vi "fgv_calibrationPos_LBVals.vi"(7 "ACtions":enum16{"Initialise", "Get", "Set"}(ring), 8 "error in (no error)":errorcluster, 11 "Calibration Pos LBVals IN":string[][](array[string])) -> (0 "error out":errorcluster, 3 "Calibration Pos LBVals  OUT":string[][](array[string]))   [LabVIEW 2020]
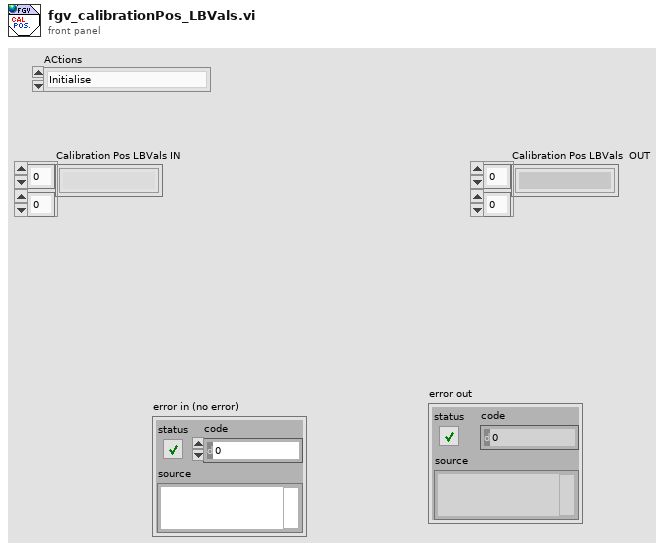
[diagram p1: front panel]
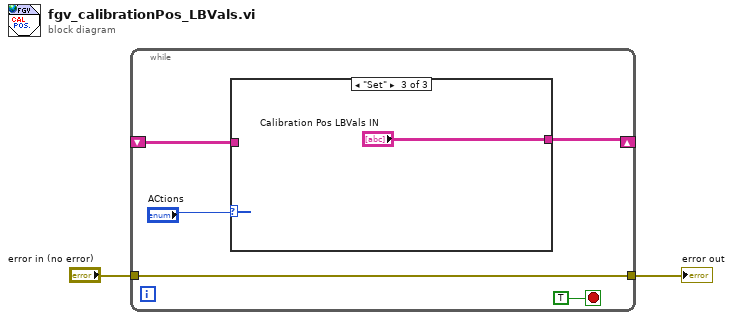
[diagram p0: block diagram]
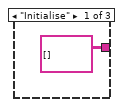
[diagram p2: hidden frame]
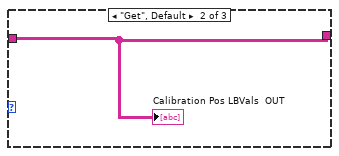
[diagram p3: hidden frame]
diagram:
  n1 = while {
    shift-right: [w6] -> _
    shift-left: _ -> [w5]
    tunnel: "error in (no error)" -> [w4]
    tunnel: [w4] -> w1
    stop <- TRUE stop-if-true
    n2 = case shown="\"Set\"" "ACtions" {
      tunnel: [string[][] [] ("Calibration Pos LBVals IN") w9 "Calibration Pos LBVals IN"] -> w6
      tunnel: w5 -> [_ w9 _]
      frame "Initialise" {
      }
      frame "Get", Default {
        "Calibration Pos LBVals  OUT" <- w9
      }
      frame "Set" {
      }
    }
  }
  "error out" <- w1
